vi "Queue Loop.vi"(11 "Queue Actor in":refnum<class "Queue Actor.lvclass">) -> (3 "Queue Actor out":refnum<class "Queue Actor.lvclass">)   [LabVIEW 2021, in "Queue Actor.lvclass"]
uses:
  Queue Actor.lvclass
  C:/git/jettl/src/Actor/Actor/Actor.lvclass
  Msg/Msg.lvclass
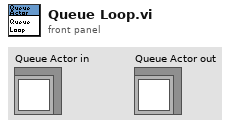
[diagram p1: front panel]
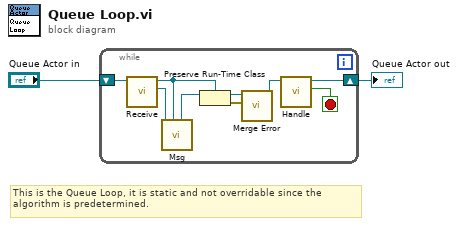
[diagram p0: block diagram]
diagram:
  # "This is the Queue Loop, it is static and not overridable since the algorithm is predetermined."
  n1 = while {
    shift-right: [w11] -> w1
    shift-left: "Queue Actor in" -> [w9]
    stop <- w10 stop-if-true
    n2 = call-dynamic "Receive.vi"("Queue Actor in"=w9) -> ("Msg"=w8:refnum<class "Msg.lvclass">, "Queue Actor out"=w3:refnum<class "Queue Actor.lvclass">)  [unwired: 9 in]
    n3 = call-dynamic "Msg.vi"("Actor in"=w3, "Msg in"=w8) -> ("Actor out"=w4:refnum<class "Actor.lvclass">)  [unwired: 9 in]
    n4 = Preserve Run-Time Class(object in=w4, 2:w3) -> (object out=w6:refnum<class "Queue Actor.lvclass">, error out=w7:errorcluster)  [unwired: 1 in]
    n5 = call-dynamic "Merge Error.vi"("Error"=w7, "Set Error in"=w6) -> ("Set Error out"=w5:refnum<class "Queue Actor.lvclass">)  [unwired: 9 in]
    n6 = call-dynamic "Handle.vi"("Actor in"=w5) -> ("Destroy?"=w10:bool, "Actor out"=w11:refnum<class "Queue Actor.lvclass">)  [unwired: 9 in]
  }
  "Queue Actor out" <- w1
